vi "Concatenate to 1D.vi"(6 "Numberofcolumns":i32, 7 "ID":i32[](array[numeric]), 8 "error in (no error)":errorcluster, 9 "Defect":bool[](array[boolean]), 10 "Terminal Data 1D":dbl[](array[numeric]), 11 "isPass":bool) -> (0 "error out":errorcluster, 3 "1D Concatenated Array":dbl[](array[numeric]))   [LabVIEW 2019, in "Zen Analytics.lvlib" / "Zen Analytics.lvclass"]
uses:
  Zen Analytics.lvclass
panel:
  out "x-y":i32
  out "OutputData 2":dbl[](array[numeric])
  out "OutputData":dbl[](array[numeric])
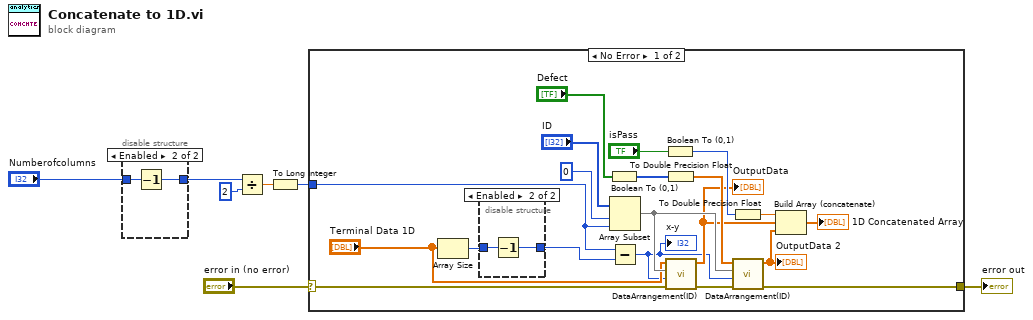
[diagram p0: block diagram]
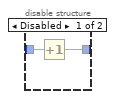
[diagram p2: hidden frame]
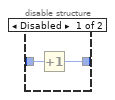
[diagram p3: hidden frame]
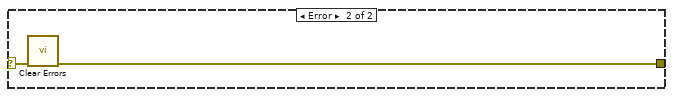
[diagram p4: hidden frame]
diagram:
  n1 = disable-structure shown="Enabled" {
    disable-tunnel: "Numberofcolumns" -> [w9 w11]
    disable-tunnel: [w8 w10] -> w1
    frame Disabled {
      n2 = Increment(x=w9) -> (x+1=w8:i32)
    }
    frame Enabled {
      n3 = Decrement(x=w11) -> (x-1=w10:i32)
    }
  }
  n4 = Divide(x=w1, y=2) -> (x/y=w3:dbl)
  n5 = To Long Integer(number=w3) -> (32bit integer=w2:i32)
  n6 = case shown="No Error" "error in (no error)" {
    selector: "error in (no error)" -> [w27 w37]
    tunnel: [w21 w36] -> w6
    tunnel: w2 -> [w15 _]
    frame No Error {
      n7 = Array Size(array="Terminal Data 1D") -> (size(s)=w14:i32)
      n8 = disable-structure shown="Enabled" {
        disable-tunnel: w14 -> [w33 w35]
        disable-tunnel: [w32 w34] -> w13
        frame Disabled {
          n9 = Increment(x=w33) -> (x+1=w32:i32)
        }
        frame Enabled {
          n10 = Decrement(x=w35) -> (x-1=w34:i32)
        }
      }
      n11 = Boolean To (0,1)(Boolean="Defect") -> (0, 1=w28:i16[])
      n12 = Array Subset(array="ID", index=0, length=w15) -> (w20:i32[])
      n13 = Subtract(x=w15, y=w13) -> (x-y=w12:i32)
      "x-y" <- w12
      n14 = Boolean To (0,1)(Boolean="isPass") -> (0, 1=w30:i16)
      n15 = To Double Precision Float(number=w28) -> (double precision float=w26:dbl[])
      n16 = call "DataArrangement(ID).vi"("error in (no error)"=w27, "y"=w12, "ID"=w20, "InputData"="Terminal Data 1D") -> ("error out"=w22:errorcluster, "OutputData"=w17:dbl[])  [unwired: 6 in]
      "OutputData" <- w17
      n17 = To Double Precision Float(number=w30) -> (double precision float=w24:dbl)
      n18 = call "DataArrangement(ID).vi"("error in (no error)"=w22, "y"=w12, "ID"=w20, "InputData"=w26) -> ("error out"=w21:errorcluster, "OutputData"=w23:dbl[])  [unwired: 6 in]
      "OutputData 2" <- w23
      n19 = Build Array (concatenate)(w24, w17, w23) -> (→"1D Concatenated Array":dbl[])
    }
    frame Error {
      n20 = call <vilib>:"Clear Errors.vi"("error in (no error)"=w37) -> ("error out"=w36:errorcluster)  [unwired: 5 in, 1 out]
    }
  }
  "error out" <- w6
